vi "Configure.vi"(8 "error in (no error)":errorcluster, 10 "Configuration":refnum<class "Form Model Configuration.lvclass">, 11 "Form Model in":refnum<class "Form Model.lvclass">) -> (0 "error out":errorcluster, 3 "Form Model out":refnum<class "Form Model.lvclass">)   [LabVIEW 2020, in "Form Model.lvlib" / "Form Model.lvclass"]
uses:
  Form Model.lvclass
  Form Model Configuration/Form Model Configuration Class/Form Model Configuration.lvclass
  Form Model.lvclass/Form Model.ctl
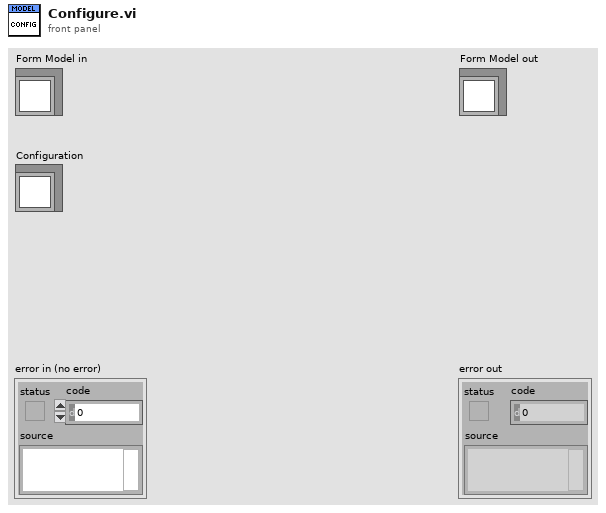
[diagram p1: front panel]
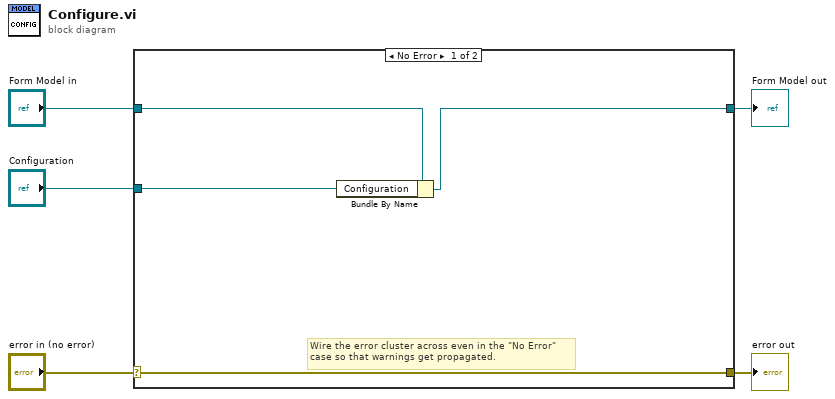
[diagram p0: block diagram]
diagram:
  n1 = case shown="No Error" "error in (no error)" {
    selector: "error in (no error)" -> [w9 w11]
    tunnel: [w9 w11] -> w4
    tunnel: [w7 w10] -> w2
    tunnel: "Form Model in" -> [w8 w10]
    tunnel: "Configuration" -> [w6 _]
    frame No Error {
      # "Wire the error cluster across even in the \"No Error\"\ncase so that warnings get propagated."
      n2 = Bundle By Name(cluster=w8, "Configuration"=w6) -> (w7:refnum<class "Form Model.lvclass">)
    }
    frame Error {
    }
  }
  "error out" <- w4
  "Form Model out" <- w2
